vi "mqttCmdCalculateByteArrayLength.vi"(5 "byteArry in":u8[](array[numeric]) format="%02x", 11 "error in (no error)":errorcluster) -> (8 "length out":u8[](array[numeric]) format="%02x", 15 "error out":errorcluster)   [LabVIEW 2015, in "mqttCmd.lvclass"]
uses:
  mqttCmd.lvclass
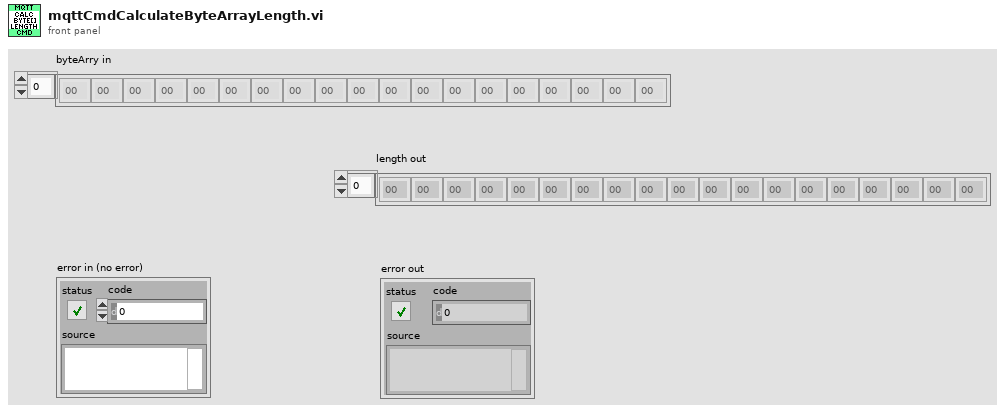
[diagram p1: front panel]
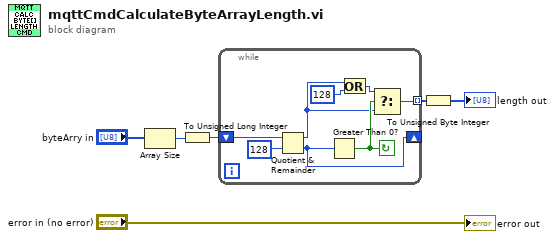
[diagram p0: block diagram]
diagram:
  n1 = Array Size(array="byteArry in") -> (size(s)=w4:i32)
  n2 = To Unsigned Long Integer(number=w4) -> (unsigned 32bit integer=w6:u32)
  n3 = while {
    shift-right: [w8] -> _
    shift-left: w6 -> [w12]
    tunnel: [w10] -> w5 mode=indexing
    stop <- w11 continue-if-true
    n4 = Quotient & Remainder(x=w12, y=u32 128) -> (x-y*floor(x/y)=w7:u32, floor(x/y)=w8:u32)
    n5 = Greater Than 0?(x=w8) -> (x > 0?=w11:bool)
    n6 = Or(x=w7, y=u32 128) -> (x .or. y?=w9:u32)
    n7 = Select(t=w9, s=w11, f=w7) -> (s? t:f=w10:u32)
  }
  n8 = To Unsigned Byte Integer(number=w5) -> (unsigned 8bit integer=→"length out":u8[])
  "error out" <- "error in (no error)"
